vi "Solve2.vi"(8 "Error In":errorcluster, 11 "object in":refnum<class "2021_6.lvclass">) -> (0 "Error Out":errorcluster, 2 "Result":u64, 3 "object out":refnum<class "2021_6.lvclass">)   [LabVIEW 2020, in "2021_6.lvclass"]
uses:
  2021_6.lvclass
  2021_6.lvclass/2021_6.ctl
panel:
  out "Numeric":i32
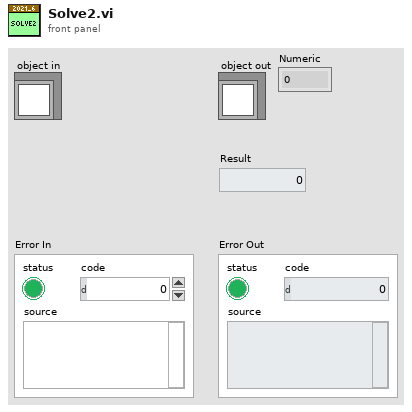
[diagram p1: front panel]
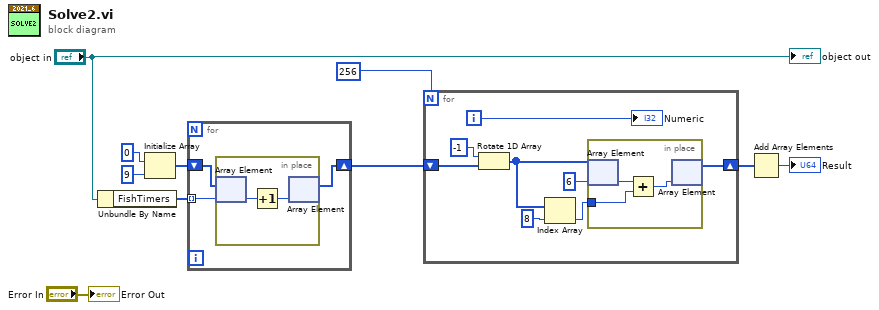
[diagram p0: block diagram]
diagram:
  n1 = Unbundle By Name("object in") -> ("FishTimers"=w1:i8[])
  n2 = Initialize Array(u64 0 ("new element/subarray"), 9 ("new element/subarray")) -> (w5:u64[])
  n3 = for {
    tunnel: w1 -> [w12] mode=indexing
    shift-right: [w11] -> w4
    shift-left: w5 -> [w13]
    n4 = in-place {
      n5 = in-place-array #1(w13, w12) -> (w15:u64)
      n6 = Increment(x=w15) -> (x+1=w14:u64)
      n7 = in-place-array #1(w14) -> (w11:u64[])  [unwired: 1 out]
    }
  }
  n8 = for {
    N: 256 -> [_]
    shift-right: [w16] -> w3
    shift-left: w4 -> [w22]
    i -> [w23]
    n9 = Rotate 1D Array(1:w22, 2:-1 ("n")) -> (0:w19:u64[])
    n10 = Index Array(array=w19, index=8) -> (element=w17:u64)
    n11 = in-place {
      in-place-border: w17 -> [w25]
      n12 = in-place-array #2(w19, 6 ("index")) -> (w26:u64)
      n13 = Add(x=w26, y=w25) -> (x+y=w24:u64)
      n14 = in-place-array #2(w24) -> (w16:u64[])  [unwired: 1 out]
    }
    "Numeric" <- w23
  }
  n15 = Add Array Elements(numeric array=w3) -> (sum=→"Result":u64)
  "Error Out" <- "Error In"
  "object out" <- "object in"
